vi "ToolBarButtonDraw_5_AutoStack.vi"(6 "Color":u32(colorbox), 8 "Focus":bool, 9 "Continuous":bool, 10 "rect":T1, 11 "Pict IN":picture) -> (3 "Pict OUT":picture)   [LabVIEW 2020, in "Sgraph_lib_V1.lvlib" / "Gviewer.lvclass"]
doc: "Draw AutoScale Stack icon in button bar"
uses:
  Gviewer.lvclass
  <vilib>/picture/picture.llb/imagedata.ctl
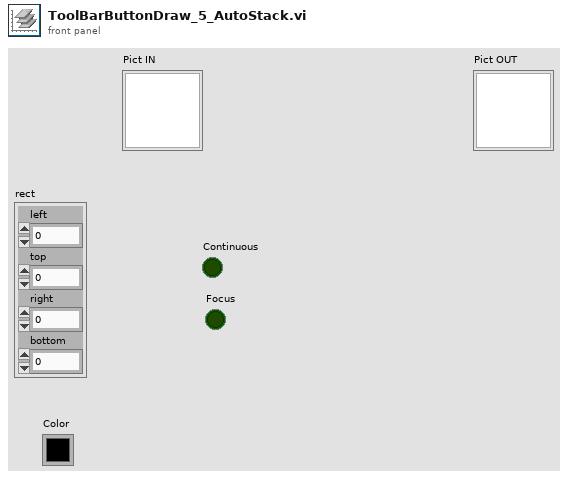
[diagram p1: front panel]
types:
  T1 = cluster{"left":i16, "top":i16, "right":i16, "bottom":i16}
  T2 = typedef "imagedata.ctl" = cluster{"image type":i32, "image depth":i32, "image":u8[], "mask":u8[], "colors":u32[], "Rectangle":cluster{"left":i16, "top":i16, "right":i16, "bottom":i16}}
  T3 = cluster{"horizontal":enum16{"left", "center", "right"}, "vertical":enum16{"top", "center", "bottom"}}
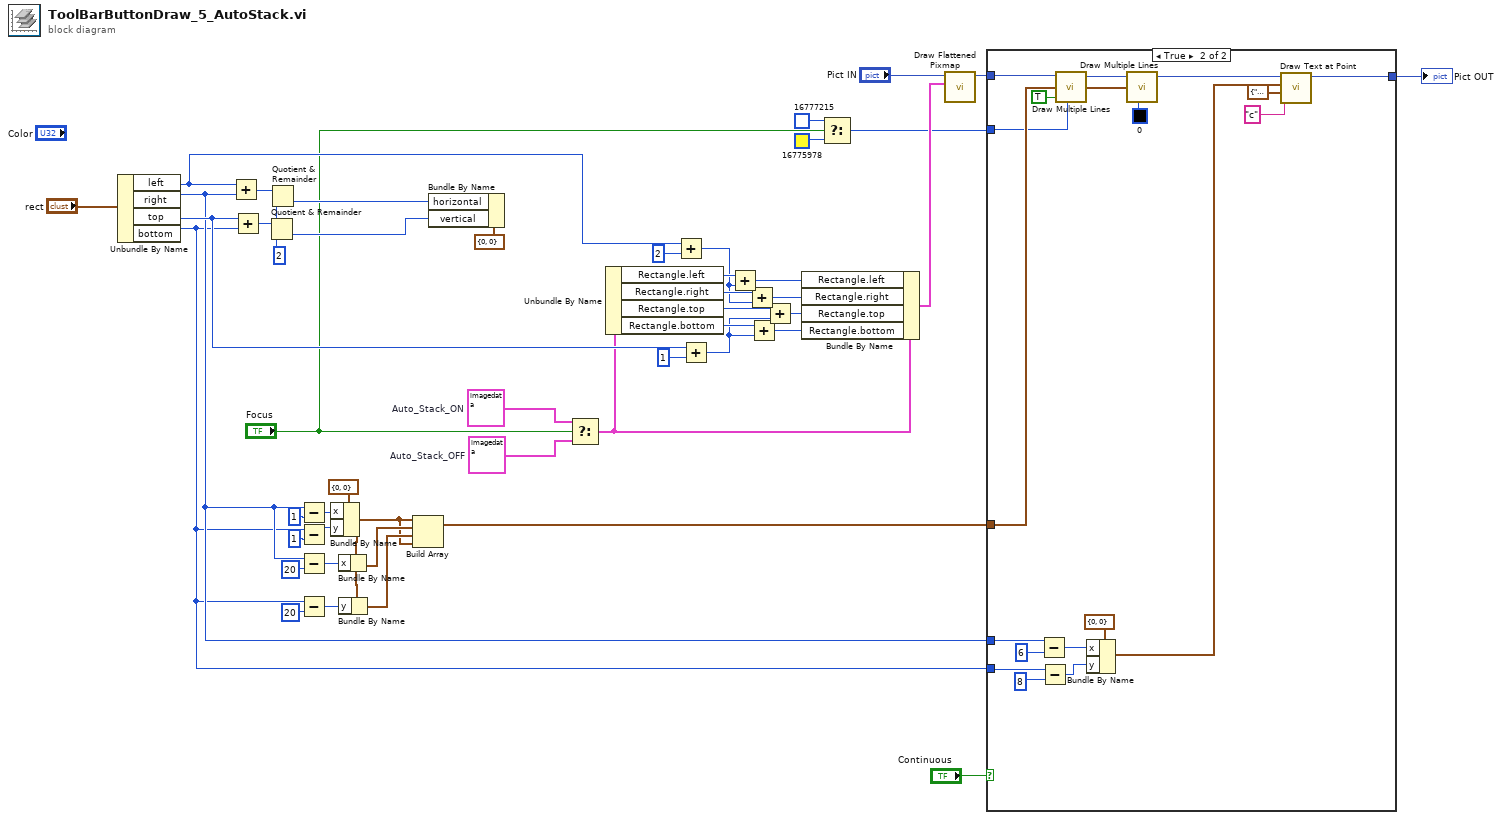
[diagram p0: block diagram]
diagram:
  w1 = T2 {"image type"=0, "image depth"=32, "image"=array[3608 elements], "mask"=[0, 0, 0, 0, 0, 0, 0, 0, 0, 127, 240, 0, 102, 24, 0, 255, 224, 0, 70, 24, 1, 255, 224, 0, 73, 36, 131, 255, 192, 0, 73, 36, 135, 255, 128, 0, 96, 195, 15, 255, 252, 0, 0, 0, 31, 255, 248, 0, 0, 0, 63, 255, 248, 0, 103, 119, 127, 255, 240, 0, 71, 119, 3, 255, 240, 0, 69, 85, 3, 255, 255, 0, 77, 221, 135, 255, 254, 0, 109, 221, 143, 255, 254, 0, 0, 0, 31, 255, 252, 0, 0, 0, 0, 255, 248, 0, 98, 34, 0, 255, 240, 0, 69, 85, 1, 255, 224, 0, 69, 85, 3, 255, 192, 0, 72, 136, 135, 255, 128, 0, 104, 136, 128, 0, 0, 0, 0, 0, 0, 0, 0, 0], "colors"=[], "Rectangle"={"left"=0, "top"=0, "right"=41, "bottom"=22}}  # Auto_Stack_ON
  w2 = T2 {"image type"=0, "image depth"=32, "image"=array[3608 elements], "mask"=[0, 0, 0, 0, 0, 0, 0, 0, 0, 127, 240, 0, 102, 24, 0, 255, 224, 0, 70, 24, 1, 255, 224, 0, 73, 36, 131, 255, 192, 0, 73, 36, 135, 255, 128, 0, 96, 195, 15, 255, 252, 0, 0, 0, 31, 255, 248, 0, 0, 0, 63, 255, 248, 0, 103, 119, 127, 255, 240, 0, 71, 119, 3, 255, 240, 0, 69, 85, 3, 255, 255, 0, 77, 221, 135, 255, 254, 0, 109, 221, 143, 255, 254, 0, 0, 0, 31, 255, 252, 0, 0, 0, 0, 255, 248, 0, 98, 34, 0, 255, 240, 0, 69, 85, 1, 255, 224, 0, 69, 85, 3, 255, 192, 0, 72, 136, 135, 255, 128, 0, 104, 136, 128, 0, 0, 0, 0, 0, 0, 0, 0, 0], "colors"=[], "Rectangle"={"left"=0, "top"=0, "right"=41, "bottom"=22}}  # Auto_Stack_OFF
  w45 = i16 2 ("y")
  n1 = Unbundle By Name("rect") -> ("left"=w29:i16, "right"=w5:i16, "top"=w20:i16, "bottom"=w4:i16)
  n2 = Add(x=w29, y=w5) -> (x+y=w47:i16)
  n3 = Add(x=w20, y=w4) -> (x+y=w46:i16)
  n4 = Quotient & Remainder(x=w46, y=w45) -> (floor(x/y)=w38:i16)  [unwired: 1 out]
  n5 = Quotient & Remainder(x=w47, y=w45) -> (floor(x/y)=w37:i16)  [unwired: 1 out]
  n6 = Subtract(x=w5, y=i16 1) -> (x-y=w42:i16)
  n7 = Subtract(x=w4, y=i16 1) -> (x-y=w15:i16)
  n8 = Subtract(x=w5, y=i16 20) -> (x-y=w40:i16)
  n9 = Subtract(x=w4, y=i16 20) -> (x-y=w14:i16)
  n10 = Bundle By Name(cluster=cluster{"x":i16, "y":i16} {"x"=0, "y"=0}, "x"=w42, "y"=w15) -> (w11:cluster{"x":i16, "y":i16})
  n11 = Bundle By Name(cluster=w11, "x"=w40) -> (w39:cluster{"x":i16, "y":i16})
  n12 = Bundle By Name(cluster=w11, "y"=w14) -> (w12:cluster{"x":i16, "y":i16})
  n13 = Build Array(w11, w39, w12, w11) -> (w18:cluster{"x":i16, "y":i16}[])
  n14 = Bundle By Name(cluster=cluster{"horizontal":i16, "vertical":i16} {"horizontal"=0, "vertical"=0} ("pixel center"), "horizontal"=w37, "vertical"=w38) -> ()  [unwired: 1 out]
  n15 = Select(t=w1, s="Focus", f=w2) -> (s? t:f=w3:T2)
  n16 = Unbundle By Name(w3) -> ("Rectangle.left"=w33:i16, "Rectangle.right"=w32:i16, "Rectangle.top"=w31:i16, "Rectangle.bottom"=w30:i16)
  n17 = Add(x=w29, y=i16 2) -> (x+y=w28:i16)
  n18 = Add(x=w20, y=i16 1) -> (x+y=w25:i16)
  n19 = Add(x=w33, y=w28) -> (x+y=w21:i16)
  n20 = Add(x=w32, y=w28) -> (x+y=w22:i16)
  n21 = Add(x=w30, y=w25) -> (x+y=w23:i16)
  n22 = Add(x=w31, y=w25) -> (x+y=w24:i16)
  n23 = Bundle By Name(cluster=w3, "Rectangle.left"=w21, "Rectangle.right"=w22, "Rectangle.top"=w24, "Rectangle.bottom"=w23) -> (w34:T2)
  n24 = Select(t=u32 16777215 ("color(black)"), s="Focus", f=u32 16775978 ("color(black)")) -> (s? t:f=w7:u32)
  n25 = call <vilib>:"Draw Flattened Pixmap.vi"("image data"=w34, "picture"="Pict IN") -> ("new picture"=w19:picture)  [unwired: 7 in]
  n26 = case shown="True" "Continuous" {
    tunnel: w19 -> [w49 w67]
    tunnel: w18 -> [_ w65]
    tunnel: [w49 w54] -> w17
    tunnel: w7 -> [_ w62]
    tunnel: w5 -> [_ w60]
    tunnel: w4 -> [_ w59]
    frame False {
    }
    frame True {
      n27 = Subtract(x=w60, y=i16 6) -> (x-y=w57:i16)
      n28 = Subtract(x=w59, y=i16 8) -> (x-y=w56:i16)
      n29 = call <vilib>:"Draw Multiple Lines.vi"("picture"=w67, "line endpoints"=w65, "fill?(F)"=TRUE, "color(black)"=w62) -> ("new picture"=w64:picture)  [unwired: 5 in]
      n30 = Bundle By Name(cluster=cluster{"x":i16, "y":i16} {"x"=0, "y"=0}, "x"=w57, "y"=w56) -> (w53:cluster{"x":i16, "y":i16})
      n31 = call <vilib>:"Draw Multiple Lines.vi"("picture"=w64, "line endpoints"=w65, "color(black)"=u32 0) -> ("new picture"=w55:picture)  [unwired: 6 in]
      n32 = call <vilib>:"Draw Text at Point.vi"("text"="c", "alignment(left, top)"=T3 {"horizontal"=enum."center", "vertical"=enum."center"}, "origin"=w53, "picture"=w55) -> ("new picture"=w54:picture)  [unwired: 6 in, 1 out]
    }
  }
  "Pict OUT" <- w17
